vi "sum_multiply.vi"(3 "Pi":T1, 5 "Pi-1":T1) -> (0 "S":cluster{"s0":bool, "s1":bool, "s2":bool}, 2 "q0":bool)   [LabVIEW 2013]
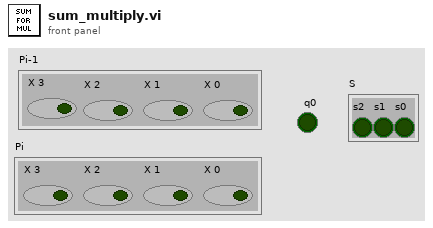
[diagram p1: front panel]
types:
  T1 = cluster{"X 0":bool, "X 1":bool, "X 2":bool, "X 3":bool}
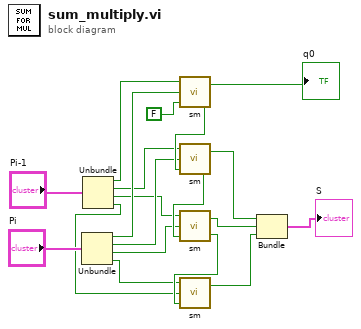
[diagram p0: block diagram]
diagram:
  n1 = Unbundle("Pi") -> ("X 0"=w13:bool, "X 1"=w10:bool, "X 2"=w8:bool, "X 3"=w7:bool)
  n2 = Unbundle("Pi-1") -> ("X 0"=w12:bool, "X 1"=w11:bool, "X 2"=w9:bool, "X 3"=w6:bool)
  n3 = call "sm.vi"("c"=FALSE, "b"=w13, "a"=w12) -> ("C"=w16:bool, "S"=→"q0":bool)
  n4 = call "sm.vi"("c"=w16, "b"=w10, "a"=w11) -> ("C"=w15:bool, "S"=w4:bool)
  n5 = call "sm.vi"("c"=w15, "b"=w8, "a"=w9) -> ("C"=w17:bool, "S"=w3:bool)
  n6 = call "sm.vi"("c"=w17, "b"=w6, "a"=w7) -> ("S"=w2:bool)  [unwired: 1 out]
  n7 = Bundle("S"=w4, "S"=w3, "S"=w2) -> (→"S":cluster{"S":bool, "S":bool, "S":bool})  [unwired: 1 in]
